vi "Update.vi"(8 "error in (no error)":errorcluster, 10 "Numeric":dbl, 11 "AbstractBattery in":refnum<class "AbstractBattery.lvclass">) -> (0 "error out":errorcluster, 3 "AbstractBattery out":refnum<class "AbstractBattery.lvclass">)   [LabVIEW 2012, in "AbstractBattery.lvclass"]
uses:
  AbstractBattery.lvclass
  AbstractBattery.lvclass/AbstractBattery.ctl
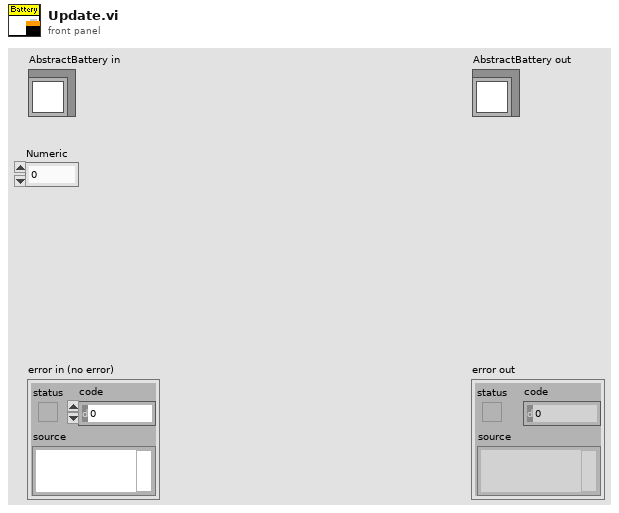
[diagram p1: front panel]
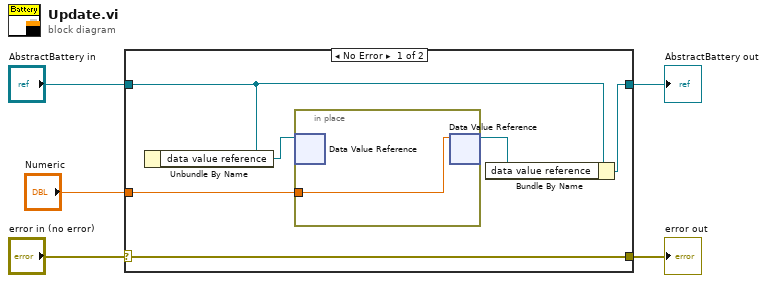
[diagram p0: block diagram]
diagram:
  n1 = case shown="No Error" "error in (no error)" {
    selector: "error in (no error)" -> [w11 w13]
    tunnel: [w11 w13] -> w4
    tunnel: [w8 w14] -> w2
    tunnel: "AbstractBattery in" -> [w6 w14]
    tunnel: "Numeric" -> [w9 _]
    frame No Error {
      n2 = Unbundle By Name(w6) -> ("data value reference"=w10:refnum<data-value>)
      n3 = in-place {
        in-place-border: w9 -> [w12]
        n4 = in-place-dvr #1(w10) -> ()  [unwired: 2 out]
        n5 = in-place-dvr #1(w12) -> (w7:refnum<data-value>)  [unwired: 1 out]
      }
      n6 = Bundle By Name(cluster=w6, "data value reference"=w7) -> (w8:refnum<class "AbstractBattery.lvclass">)
    }
    frame Error {
    }
  }
  "error out" <- w4
  "AbstractBattery out" <- w2
